vi "Spindle_load_RT (SubVI).vi"(9 "?":T1, 10 "concatenated string 4":string, 11 "String":string) -> (0 "error out":errorcluster, 3 "output cluster":T1, 4 "empty? 2":bool)   [LabVIEW 2017]
uses:
  MT_connect_data.ctl
  <vilib>/regexp/Match Regular Expression.xnode
  <vilib>/addons/internet/NI_InternetTK_Core_VIs.lvlib
panel:
  out "concatenated string 6":string
  out "concatenated string 5":string
  out "error out 2":errorcluster
  out "empty? 3":bool
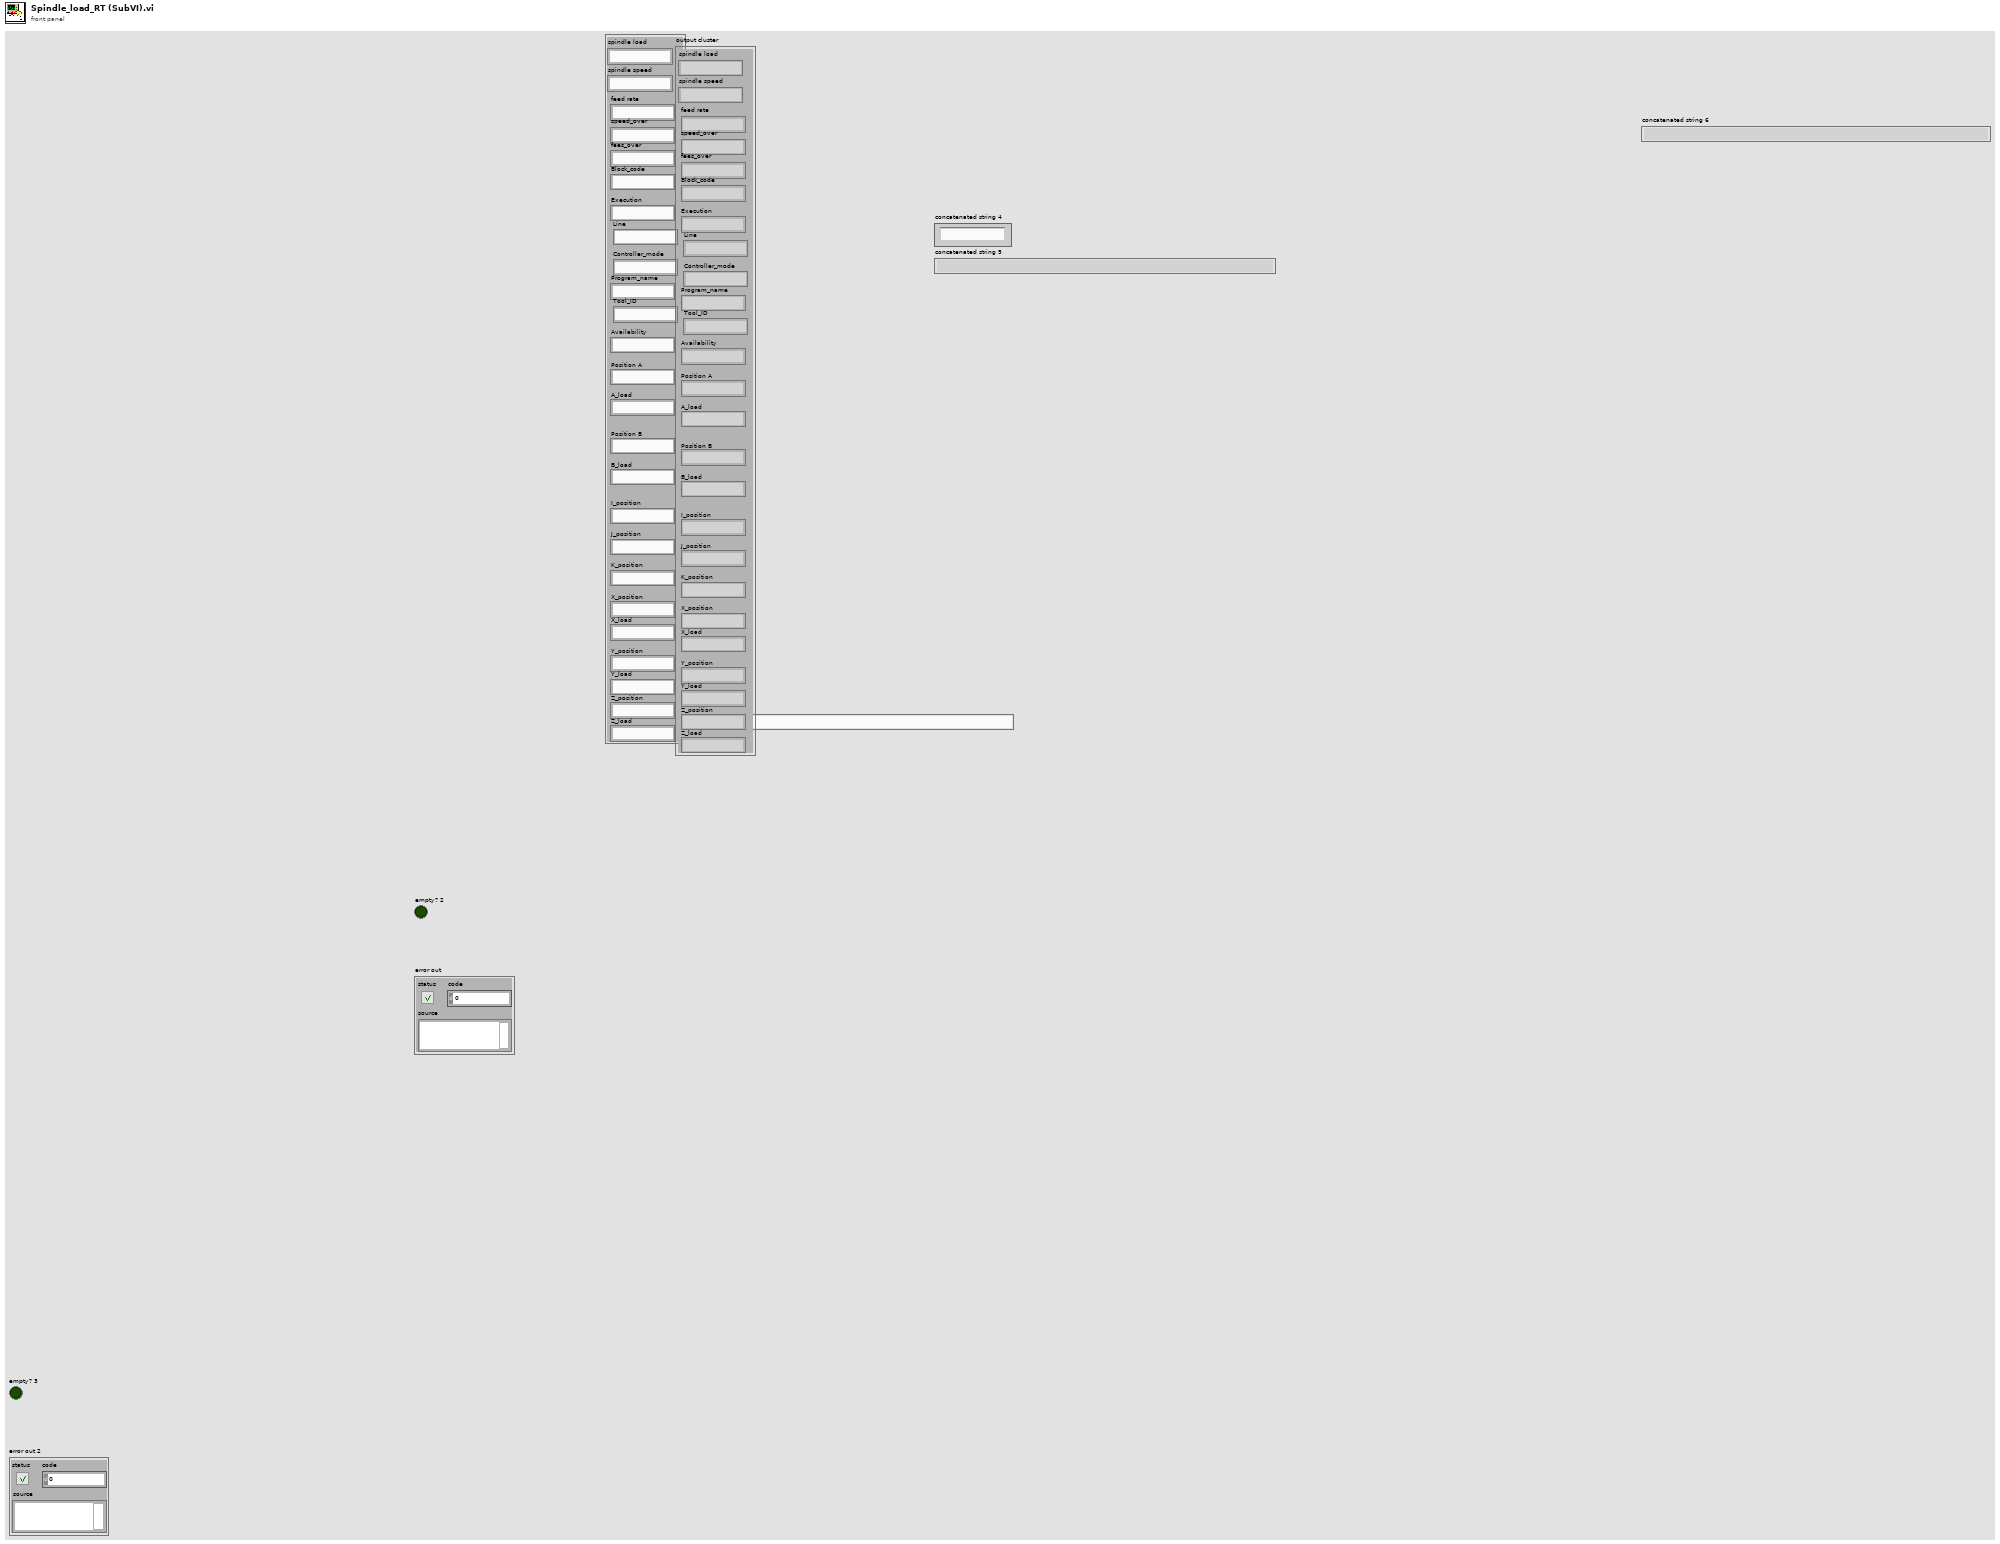
[diagram p1: front panel]
types:
  T1 = typedef "MT_connect_data.ctl" = cluster{"spindle load ":string, "spindle speed ":string, "feed rate":string, "speed_over":string, "fees_over":string, "Block_code":string, "Execution":string, "Line":string, "Controller_mode":string, "Program_name":string, "Tool_ID":string, "Availability":string, "Position A":string, "A_load":string, "Position B":string, "B_load":string, "I_position":string, "J_position":string, "K_position":string, "X_position":string, "X_load":string, "Y_position":string, "Y_load":string, "Z_position":string, "Z_load":string}
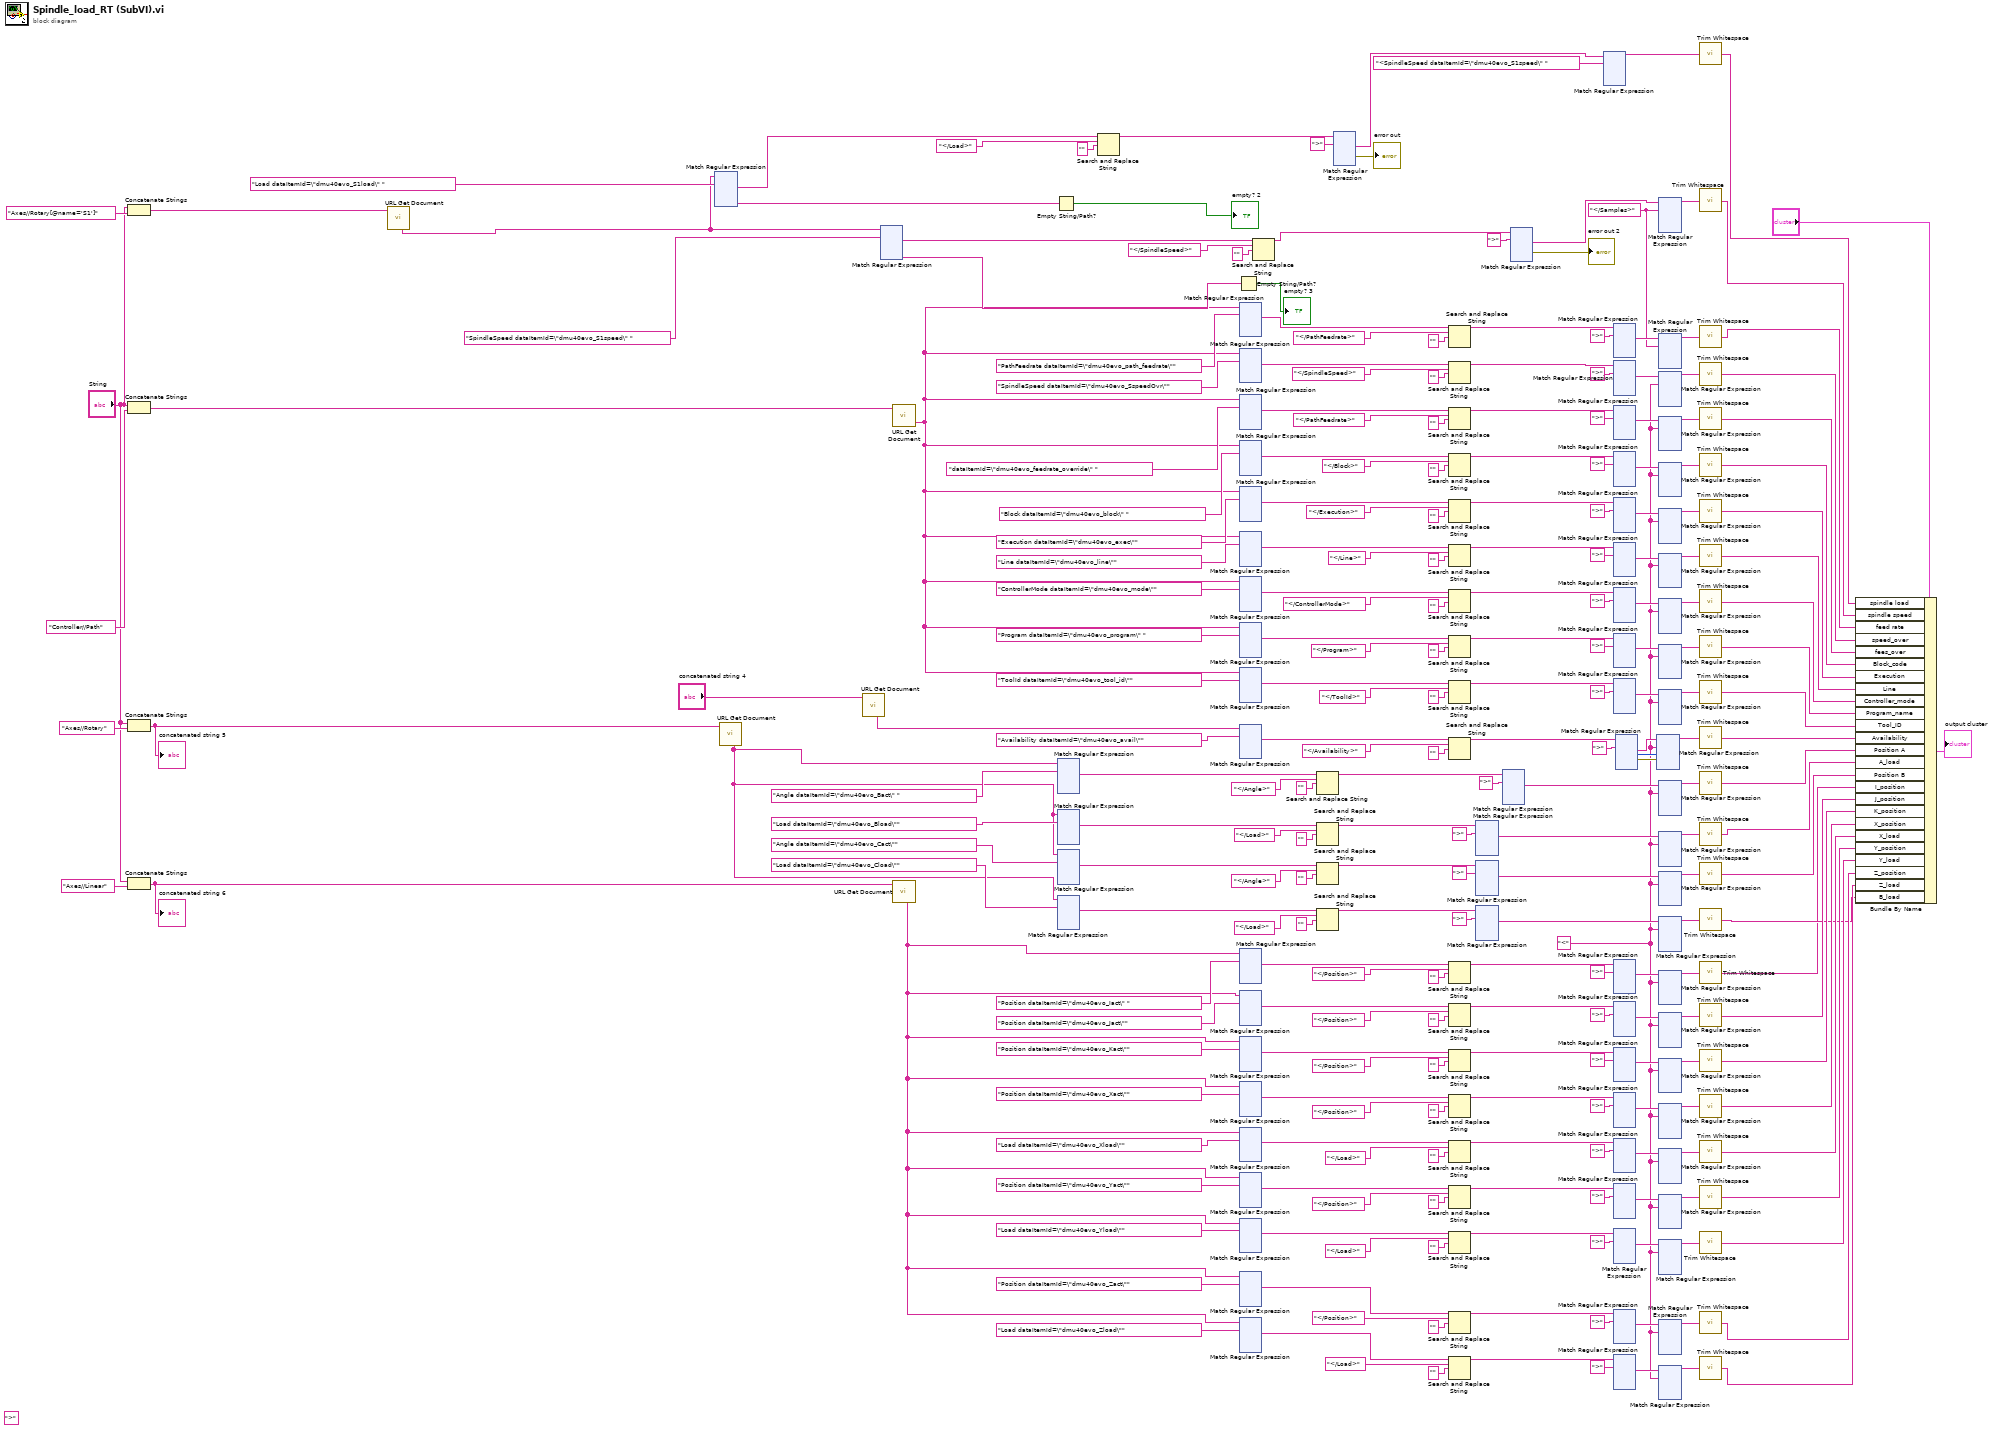
[diagram p0: block diagram]
diagram:
  w5 = "<" ("string")
  w56 = "</Samples>" ("string")
  (unwired) ">" ("string")
  n1 = Concatenate Strings("String", "Axes//Rotary[@name='S1']" ("string")) -> (w247:string)
  n2 = Concatenate Strings("String", "Controller//Path" ("string")) -> (w228:string)
  n3 = Concatenate Strings("String", "Axes//Rotary" ("string")) -> (w128:string)
  "concatenated string 5" <- w128
  n4 = Concatenate Strings("String", "Axes//Linear" ("string")) -> (w127:string)
  "concatenated string 6" <- w127
  n5 = call <vilib>:"URL Get Document.vi"("URL"=w247) -> ("content"=w233:string)  [unwired: 6 in, 4 out]
  n6 = xnode "Match Regular Expression"("input string"=w233, "regular expression"="Load dataItemId=\"dmu40evo_S1load\" ") -> ("after match"=w244:string, "submatch 1"=w246:string)  [unwired: 4 in, 4 out]
  n7 = call <vilib>:"URL Get Document.vi"("URL"=w128) -> ("content"=w132:string)  [unwired: 6 in, 4 out]
  n8 = call <vilib>:"URL Get Document.vi"("URL"="concatenated string 4") -> ("content"=w163:string)  [unwired: 6 in, 4 out]
  n9 = xnode "Match Regular Expression"("input string"=w233, "regular expression"="SpindleSpeed dataItemId=\"dmu40evo_S1speed\" ") -> ("after match"=w235:string, "submatch 1"=w237:string)  [unwired: 4 in, 4 out]
  n10 = call <vilib>:"URL Get Document.vi"("URL"=w228) -> ("content"=w1:string)  [unwired: 6 in, 4 out]
  n11 = call <vilib>:"URL Get Document.vi"("URL"=w127) -> ("content"=w71:string)  [unwired: 6 in, 4 out]
  n12 = Empty String/Path?(string/path=w246) -> (empty?=→"empty? 2":bool)
  n13 = xnode "Match Regular Expression"("input string"=w132, "regular expression"="Angle dataItemId=\"dmu40evo_Bact\" ") -> ("after match"=w156:string)  [unwired: 4 in, 5 out]
  n14 = xnode "Match Regular Expression"("input string"=w132, "regular expression"="Load dataItemId=\"dmu40evo_Bload\"") -> ("after match"=w146:string)  [unwired: 4 in, 5 out]
  n15 = xnode "Match Regular Expression"("input string"=w132, "regular expression"="Angle dataItemId=\"dmu40evo_Cact\"") -> ("after match"=w134:string)  [unwired: 4 in, 5 out]
  n16 = xnode "Match Regular Expression"("input string"=w132, "regular expression"="Load dataItemId=\"dmu40evo_Cload\"") -> ("after match"=w143:string)  [unwired: 4 in, 5 out]
  n17 = Search and Replace String(input string=w244, search string="</Load>" ("string"), replace string="" ("string")) -> (result string=w243:string)  [unwired: 5 in, 3 out]
  n18 = Empty String/Path?(string/path=w237) -> (empty?=→"empty? 3":bool)
  n19 = xnode "Match Regular Expression"("input string"=w1, "regular expression"="PathFeedrate dataItemId=\"dmu40evo_path_feedrate\"") -> ("after match"=w226:string)  [unwired: 4 in, 5 out]
  n20 = xnode "Match Regular Expression"("input string"=w1, "regular expression"="SpindleSpeed dataItemId=\"dmu40evo_SspeedOvr\"") -> ("after match"=w214:string)  [unwired: 4 in, 5 out]
  n21 = xnode "Match Regular Expression"("input string"=w1, "regular expression"="dataItemId=\"dmu40evo_feedrate_override\" ") -> ("after match"=w213:string)  [unwired: 4 in, 5 out]
  n22 = xnode "Match Regular Expression"("input string"=w1, "regular expression"="Block dataItemId=\"dmu40evo_block\" ") -> ("after match"=w200:string)  [unwired: 4 in, 5 out]
  n23 = xnode "Match Regular Expression"("input string"=w1, "regular expression"="Execution dataItemId=\"dmu40evo_exec\"") -> ("after match"=w192:string)  [unwired: 4 in, 5 out]
  n24 = xnode "Match Regular Expression"("input string"=w1, "regular expression"="Line dataItemId=\"dmu40evo_line\"") -> ("after match"=w191:string)  [unwired: 4 in, 5 out]
  n25 = xnode "Match Regular Expression"("input string"=w1, "regular expression"="ControllerMode dataItemId=\"dmu40evo_mode\"") -> ("after match"=w187:string)  [unwired: 4 in, 5 out]
  n26 = xnode "Match Regular Expression"("input string"=w1, "regular expression"="Program dataItemId=\"dmu40evo_program\" ") -> ("after match"=w178:string)  [unwired: 4 in, 5 out]
  n27 = xnode "Match Regular Expression"("input string"=w1, "regular expression"="ToolId dataItemId=\"dmu40evo_tool_id\"") -> ("after match"=w175:string)  [unwired: 4 in, 5 out]
  n28 = xnode "Match Regular Expression"("input string"=w163, "regular expression"="Availability dataItemId=\"dmu40evo_avail\"") -> ("after match"=w166:string)  [unwired: 4 in, 5 out]
  n29 = xnode "Match Regular Expression"("input string"=w71, "regular expression"="Position dataItemId=\"dmu40evo_Iact\" ") -> ("after match"=w121:string)  [unwired: 4 in, 5 out]
  n30 = xnode "Match Regular Expression"("input string"=w71, "regular expression"="Position dataItemId=\"dmu40evo_Jact\"") -> ("after match"=w118:string)  [unwired: 4 in, 5 out]
  n31 = xnode "Match Regular Expression"("input string"=w71, "regular expression"="Position dataItemId=\"dmu40evo_Kact\"") -> ("after match"=w109:string)  [unwired: 4 in, 5 out]
  n32 = xnode "Match Regular Expression"("input string"=w71, "regular expression"="Position dataItemId=\"dmu40evo_Xact\"") -> ("after match"=w94:string)  [unwired: 4 in, 5 out]
  n33 = xnode "Match Regular Expression"("input string"=w71, "regular expression"="Load dataItemId=\"dmu40evo_Xload\"") -> ("after match"=w97:string)  [unwired: 4 in, 5 out]
  n34 = xnode "Match Regular Expression"("input string"=w71, "regular expression"="Position dataItemId=\"dmu40evo_Yact\"") -> ("after match"=w106:string)  [unwired: 4 in, 5 out]
  n35 = xnode "Match Regular Expression"("input string"=w71, "regular expression"="Load dataItemId=\"dmu40evo_Yload\"") -> ("after match"=w85:string)  [unwired: 4 in, 5 out]
  n36 = xnode "Match Regular Expression"("input string"=w71, "regular expression"="Position dataItemId=\"dmu40evo_Zact\"") -> ("after match"=w73:string)  [unwired: 4 in, 5 out]
  n37 = xnode "Match Regular Expression"("input string"=w71, "regular expression"="Load dataItemId=\"dmu40evo_Zload\"") -> ("after match"=w82:string)  [unwired: 4 in, 5 out]
  n38 = Search and Replace String(input string=w235, search string="</SpindleSpeed>" ("string"), replace string="" ("string")) -> (result string=w234:string)  [unwired: 5 in, 3 out]
  n39 = Search and Replace String(input string=w156, search string="</Angle>" ("string"), replace string="" ("string")) -> (result string=w157:string)  [unwired: 5 in, 3 out]
  n40 = Search and Replace String(input string=w146, search string="</Load>" ("string"), replace string="" ("string")) -> (result string=w145:string)  [unwired: 5 in, 3 out]
  n41 = Search and Replace String(input string=w134, search string="</Angle>" ("string"), replace string="" ("string")) -> (result string=w133:string)  [unwired: 5 in, 3 out]
  n42 = Search and Replace String(input string=w143, search string="</Load>" ("string"), replace string="" ("string")) -> (result string=w144:string)  [unwired: 5 in, 3 out]
  n43 = xnode "Match Regular Expression"("input string"=w243, "regular expression"=">" ("string")) -> ("after match"=w60:string, "error out"=→"error out":errorcluster)  [unwired: 4 in, 4 out]
  n44 = Search and Replace String(input string=w226, search string="</PathFeedrate>" ("string"), replace string="" ("string")) -> (result string=w221:string)  [unwired: 5 in, 3 out]
  n45 = Search and Replace String(input string=w214, search string="</SpindleSpeed>" ("string"), replace string="" ("string")) -> (result string=w219:string)  [unwired: 5 in, 3 out]
  n46 = Search and Replace String(input string=w213, search string="</PathFeedrate>" ("string"), replace string="" ("string")) -> (result string=w208:string)  [unwired: 5 in, 3 out]
  n47 = Search and Replace String(input string=w200, search string="</Block>" ("string"), replace string="" ("string")) -> (result string=w205:string)  [unwired: 5 in, 3 out]
  n48 = Search and Replace String(input string=w192, search string="</Execution>" ("string"), replace string="" ("string")) -> (result string=w190:string)  [unwired: 5 in, 3 out]
  n49 = Search and Replace String(input string=w191, search string="</Line>" ("string"), replace string="" ("string")) -> (result string=w189:string)  [unwired: 5 in, 3 out]
  n50 = Search and Replace String(input string=w187, search string="</ControllerMode>" ("string"), replace string="" ("string")) -> (result string=w188:string)  [unwired: 5 in, 3 out]
  n51 = Search and Replace String(input string=w178, search string="</Program>" ("string"), replace string="" ("string")) -> (result string=w177:string)  [unwired: 5 in, 3 out]
  n52 = Search and Replace String(input string=w175, search string="</ToolId>" ("string"), replace string="" ("string")) -> (result string=w176:string)  [unwired: 5 in, 3 out]
  n53 = Search and Replace String(input string=w166, search string="</Availability>" ("string"), replace string="" ("string")) -> (result string=w165:string)  [unwired: 5 in, 3 out]
  n54 = Search and Replace String(input string=w121, search string="</Position>" ("string"), replace string="" ("string")) -> (result string=w120:string)  [unwired: 5 in, 3 out]
  n55 = Search and Replace String(input string=w118, search string="</Position>" ("string"), replace string="" ("string")) -> (result string=w119:string)  [unwired: 5 in, 3 out]
  n56 = Search and Replace String(input string=w109, search string="</Position>" ("string"), replace string="" ("string")) -> (result string=w108:string)  [unwired: 5 in, 3 out]
  n57 = Search and Replace String(input string=w94, search string="</Position>" ("string"), replace string="" ("string")) -> (result string=w95:string)  [unwired: 5 in, 3 out]
  n58 = Search and Replace String(input string=w97, search string="</Load>" ("string"), replace string="" ("string")) -> (result string=w96:string)  [unwired: 5 in, 3 out]
  n59 = Search and Replace String(input string=w106, search string="</Position>" ("string"), replace string="" ("string")) -> (result string=w107:string)  [unwired: 5 in, 3 out]
  n60 = Search and Replace String(input string=w85, search string="</Load>" ("string"), replace string="" ("string")) -> (result string=w84:string)  [unwired: 5 in, 3 out]
  n61 = Search and Replace String(input string=w73, search string="</Position>" ("string"), replace string="" ("string")) -> (result string=w72:string)  [unwired: 5 in, 3 out]
  n62 = Search and Replace String(input string=w82, search string="</Load>" ("string"), replace string="" ("string")) -> (result string=w83:string)  [unwired: 5 in, 3 out]
  n63 = xnode "Match Regular Expression"("input string"=w145, "regular expression"=">" ("string")) -> ("after match"=w36:string)  [unwired: 4 in, 5 out]
  n64 = xnode "Match Regular Expression"("input string"=w133, "regular expression"=">" ("string")) -> ("after match"=w35:string)  [unwired: 4 in, 5 out]
  n65 = xnode "Match Regular Expression"("input string"=w144, "regular expression"=">" ("string")) -> ("after match"=w34:string)  [unwired: 4 in, 5 out]
  n66 = xnode "Match Regular Expression"("input string"=w157, "regular expression"=">" ("string")) -> ("after match"=w24:string)  [unwired: 4 in, 5 out]
  n67 = xnode "Match Regular Expression"("input string"=w234, "regular expression"=">" ("string")) -> ("after match"=w59:string, "error out"=→"error out 2":errorcluster)  [unwired: 4 in, 4 out]
  n68 = xnode "Match Regular Expression"("input string"=w60, "regular expression"="<SpindleSpeed dataItemId=\"dmu40evo_S1speed\" ") -> ("before match"=w61:string)  [unwired: 4 in, 5 out]
  n69 = xnode "Match Regular Expression"("input string"=w221, "regular expression"=">" ("string")) -> ("after match"=w57:string)  [unwired: 4 in, 5 out]
  n70 = xnode "Match Regular Expression"("input string"=w219, "regular expression"=">" ("string")) -> ("after match"=w50:string)  [unwired: 4 in, 5 out]
  n71 = xnode "Match Regular Expression"("input string"=w208, "regular expression"=">" ("string")) -> ("after match"=w6:string)  [unwired: 4 in, 5 out]
  n72 = xnode "Match Regular Expression"("input string"=w205, "regular expression"=">" ("string")) -> ("after match"=w9:string)  [unwired: 4 in, 5 out]
  n73 = xnode "Match Regular Expression"("input string"=w190, "regular expression"=">" ("string")) -> ("after match"=w52:string)  [unwired: 4 in, 5 out]
  n74 = xnode "Match Regular Expression"("input string"=w189, "regular expression"=">" ("string")) -> ("after match"=w48:string)  [unwired: 4 in, 5 out]
  n75 = xnode "Match Regular Expression"("input string"=w188, "regular expression"=">" ("string")) -> ("after match"=w46:string)  [unwired: 4 in, 5 out]
  n76 = xnode "Match Regular Expression"("input string"=w177, "regular expression"=">" ("string")) -> ("after match"=w40:string)  [unwired: 4 in, 5 out]
  n77 = xnode "Match Regular Expression"("input string"=w176, "regular expression"=">" ("string")) -> ("after match"=w39:string)  [unwired: 4 in, 5 out]
  n78 = xnode "Match Regular Expression"("input string"=w120, "regular expression"=">" ("string")) -> ("after match"=w33:string)  [unwired: 4 in, 5 out]
  n79 = xnode "Match Regular Expression"("input string"=w119, "regular expression"=">" ("string")) -> ("after match"=w32:string)  [unwired: 4 in, 5 out]
  n80 = xnode "Match Regular Expression"("input string"=w108, "regular expression"=">" ("string")) -> ("after match"=w31:string)  [unwired: 4 in, 5 out]
  n81 = xnode "Match Regular Expression"("input string"=w95, "regular expression"=">" ("string")) -> ("after match"=w30:string)  [unwired: 4 in, 5 out]
  n82 = xnode "Match Regular Expression"("input string"=w96, "regular expression"=">" ("string")) -> ("after match"=w29:string)  [unwired: 4 in, 5 out]
  n83 = xnode "Match Regular Expression"("input string"=w107, "regular expression"=">" ("string")) -> ("after match"=w28:string)  [unwired: 4 in, 5 out]
  n84 = xnode "Match Regular Expression"("input string"=w84, "regular expression"=">" ("string")) -> ("after match"=w27:string)  [unwired: 4 in, 5 out]
  n85 = xnode "Match Regular Expression"("input string"=w72, "regular expression"=">" ("string")) -> ("after match"=w26:string)  [unwired: 4 in, 5 out]
  n86 = xnode "Match Regular Expression"("input string"=w83, "regular expression"=">" ("string")) -> ("after match"=w25:string)  [unwired: 4 in, 5 out]
  n87 = xnode "Match Regular Expression"("input string"=w165, "regular expression"=">" ("string")) -> ("after match"=w38:string, "offset past match"=w42:i32, "error out"=w41:errorcluster)  [unwired: 4 in, 3 out]
  n88 = xnode "Match Regular Expression"("input string"=w38, "regular expression"=w5, "offset (0)"=w42, "error in"=w41) -> ("before match"=w23:string)  [unwired: 2 in, 5 out]
  n89 = xnode "Match Regular Expression"("input string"=w59, "regular expression"=w56) -> ("before match"=w58:string)  [unwired: 4 in, 5 out]
  n90 = xnode "Match Regular Expression"("input string"=w57, "regular expression"=w56) -> ("before match"=w55:string)  [unwired: 4 in, 5 out]
  n91 = xnode "Match Regular Expression"("input string"=w50, "regular expression"=w5) -> ("before match"=w54:string)  [unwired: 4 in, 5 out]
  n92 = xnode "Match Regular Expression"("input string"=w6, "regular expression"=w5) -> ("before match"=w7:string)  [unwired: 4 in, 5 out]
  n93 = xnode "Match Regular Expression"("input string"=w9, "regular expression"=w5) -> ("before match"=w8:string)  [unwired: 4 in, 5 out]
  n94 = xnode "Match Regular Expression"("input string"=w52, "regular expression"=w5) -> ("before match"=w51:string)  [unwired: 4 in, 5 out]
  n95 = xnode "Match Regular Expression"("input string"=w48, "regular expression"=w5) -> ("before match"=w47:string)  [unwired: 4 in, 5 out]
  n96 = xnode "Match Regular Expression"("input string"=w46, "regular expression"=w5) -> ("before match"=w45:string)  [unwired: 4 in, 5 out]
  n97 = xnode "Match Regular Expression"("input string"=w40, "regular expression"=w5) -> ("before match"=w44:string)  [unwired: 4 in, 5 out]
  n98 = xnode "Match Regular Expression"("input string"=w39, "regular expression"=w5) -> ("before match"=w43:string)  [unwired: 4 in, 5 out]
  n99 = xnode "Match Regular Expression"("input string"=w24, "regular expression"=w5) -> ("before match"=w22:string)  [unwired: 4 in, 5 out]
  n100 = xnode "Match Regular Expression"("input string"=w36, "regular expression"=w5) -> ("before match"=w21:string)  [unwired: 4 in, 5 out]
  n101 = xnode "Match Regular Expression"("input string"=w35, "regular expression"=w5) -> ("before match"=w20:string)  [unwired: 4 in, 5 out]
  n102 = xnode "Match Regular Expression"("input string"=w34, "regular expression"=w5) -> ("before match"=w19:string)  [unwired: 4 in, 5 out]
  n103 = xnode "Match Regular Expression"("input string"=w33, "regular expression"=w5) -> ("before match"=w18:string)  [unwired: 4 in, 5 out]
  n104 = xnode "Match Regular Expression"("input string"=w32, "regular expression"=w5) -> ("before match"=w17:string)  [unwired: 4 in, 5 out]
  n105 = xnode "Match Regular Expression"("input string"=w31, "regular expression"=w5) -> ("before match"=w16:string)  [unwired: 4 in, 5 out]
  n106 = xnode "Match Regular Expression"("input string"=w30, "regular expression"=w5) -> ("before match"=w15:string)  [unwired: 4 in, 5 out]
  n107 = xnode "Match Regular Expression"("input string"=w29, "regular expression"=w5) -> ("before match"=w14:string)  [unwired: 4 in, 5 out]
  n108 = xnode "Match Regular Expression"("input string"=w28, "regular expression"=w5) -> ("before match"=w13:string)  [unwired: 4 in, 5 out]
  n109 = xnode "Match Regular Expression"("input string"=w27, "regular expression"=w5) -> ("before match"=w12:string)  [unwired: 4 in, 5 out]
  n110 = xnode "Match Regular Expression"("input string"=w26, "regular expression"=w5) -> ("before match"=w11:string)  [unwired: 4 in, 5 out]
  n111 = xnode "Match Regular Expression"("input string"=w25, "regular expression"=w5) -> ("before match"=w10:string)  [unwired: 4 in, 5 out]
  n112 = call <vilib>:"Trim Whitespace.vi"("string"=w61) -> ("trimmed string"=w231:string)  [unwired: 1 in]
  n113 = call <vilib>:"Trim Whitespace.vi"("string"=w58) -> ("trimmed string"=w230:string)  [unwired: 1 in]
  n114 = call <vilib>:"Trim Whitespace.vi"("string"=w55) -> ("trimmed string"=w220:string)  [unwired: 1 in]
  n115 = call <vilib>:"Trim Whitespace.vi"("string"=w54) -> ("trimmed string"=w207:string)  [unwired: 1 in]
  n116 = call <vilib>:"Trim Whitespace.vi"("string"=w7) -> ("trimmed string"=w206:string)  [unwired: 1 in]
  n117 = call <vilib>:"Trim Whitespace.vi"("string"=w8) -> ("trimmed string"=w4:string)  [unwired: 1 in]
  n118 = call <vilib>:"Trim Whitespace.vi"("string"=w51) -> ("trimmed string"=w162:string)  [unwired: 1 in]
  n119 = call <vilib>:"Trim Whitespace.vi"("string"=w47) -> ("trimmed string"=w49:string)  [unwired: 1 in]
  n120 = call <vilib>:"Trim Whitespace.vi"("string"=w45) -> ("trimmed string"=w161:string)  [unwired: 1 in]
  n121 = call <vilib>:"Trim Whitespace.vi"("string"=w44) -> ("trimmed string"=w160:string)  [unwired: 1 in]
  n122 = call <vilib>:"Trim Whitespace.vi"("string"=w43) -> ("trimmed string"=w159:string)  [unwired: 1 in]
  n123 = call <vilib>:"Trim Whitespace.vi"("string"=w23) -> ("trimmed string"=w158:string)  [unwired: 1 in]
  n124 = call <vilib>:"Trim Whitespace.vi"("string"=w22) -> ("trimmed string"=w131:string)  [unwired: 1 in]
  n125 = call <vilib>:"Trim Whitespace.vi"("string"=w21) -> ("trimmed string"=w37:string)  [unwired: 1 in]
  n126 = call <vilib>:"Trim Whitespace.vi"("string"=w20) -> ("trimmed string"=w130:string)  [unwired: 1 in]
  n127 = call <vilib>:"Trim Whitespace.vi"("string"=w19) -> ("trimmed string"=w3:string)  [unwired: 1 in]
  n128 = call <vilib>:"Trim Whitespace.vi"("string"=w18) -> ("trimmed string"=w2:string)  [unwired: 1 in]
  n129 = call <vilib>:"Trim Whitespace.vi"("string"=w17) -> ("trimmed string"=w70:string)  [unwired: 1 in]
  n130 = call <vilib>:"Trim Whitespace.vi"("string"=w16) -> ("trimmed string"=w69:string)  [unwired: 1 in]
  n131 = call <vilib>:"Trim Whitespace.vi"("string"=w15) -> ("trimmed string"=w68:string)  [unwired: 1 in]
  n132 = call <vilib>:"Trim Whitespace.vi"("string"=w14) -> ("trimmed string"=w67:string)  [unwired: 1 in]
  n133 = call <vilib>:"Trim Whitespace.vi"("string"=w13) -> ("trimmed string"=w66:string)  [unwired: 1 in]
  n134 = call <vilib>:"Trim Whitespace.vi"("string"=w12) -> ("trimmed string"=w65:string)  [unwired: 1 in]
  n135 = call <vilib>:"Trim Whitespace.vi"("string"=w11) -> ("trimmed string"=w64:string)  [unwired: 1 in]
  n136 = call <vilib>:"Trim Whitespace.vi"("string"=w10) -> ("trimmed string"=w63:string)  [unwired: 1 in]
  n137 = Bundle By Name(cluster="?", "spindle load"=w231, "spindle speed"=w230, "feed rate"=w220, "speed_over"=w207, "fees_over"=w206, "Block_code"=w4, "Execution"=w162, "Line"=w49, "Controller_mode"=w161, "Program_name"=w160, "Tool_ID"=w159, "Availability"=w158, "Position A"=w131, "A_load"=w37, "Position B"=w130, "I_position"=w2, "J_position"=w70, "K_position"=w69, "X_position"=w68, "X_load"=w67, "Y_position"=w66, "Y_load"=w65, "Z_position"=w64, "Z_load"=w63, "B_load"=w3) -> (→"output cluster":T1)
